vi "Local Variables.vi"() -> ()   [LabVIEW 2012]
panel:
  in  "停止按钮":bool
  out "图表2":dbl(graph)
  out "图表1":dbl(graph)
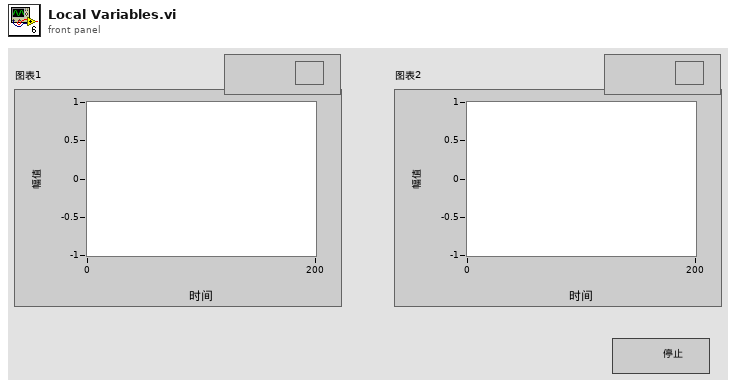
[diagram p1: front panel]
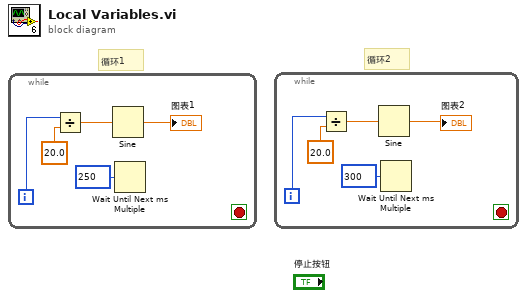
[diagram p0: block diagram]
diagram:
  # "循环1"
  # "循环2"
  n1 = while "Loop 1" {
    i -> [w5]
    stop <- _ stop-if-true
    n2 = Divide ("除")(x=w5, y=20.0) -> (x/y=w3:dbl)
    n3 = Sine ("正弦")(x=w3) -> (sin(x)=→"图表1":dbl)
    n4 = Wait Until Next ms Multiple ("等待下一个整数倍毫秒")(millisecond multiple=u32 250 ("毫秒倍数")) -> ()  [unwired: 1 out]
  }
  n5 = while "Loop 2" {
    i -> [w10]
    stop <- _ stop-if-true
    n6 = Divide ("除")(x=w10, y=20.0) -> (x/y=w8:dbl)
    n7 = Sine ("正弦")(x=w8) -> (sin(x)=→"图表2":dbl)
    n8 = Wait Until Next ms Multiple ("等待下一个整数倍毫秒")(millisecond multiple=u32 300 ("毫秒倍数")) -> ()  [unwired: 1 out]
  }
